vi "DQBuf.vi"(0 "nInputHandle":u64, 2 "nTimeOut":u32, 5 "error in (no error)":errorcluster) -> (14 "nOutputHandle":u64, 15 "ImgBuf":u8[](array[numeric]), 16 "ppFrameBuffer":u64, 17 "Dst":T1, 18 "GX_STATUS":i32, 19 "error out":errorcluster)   [LabVIEW 2016, in "GxLVLib.lvlib"]
uses:
  GxLVLib.lvlib
  GxIAPI.dll
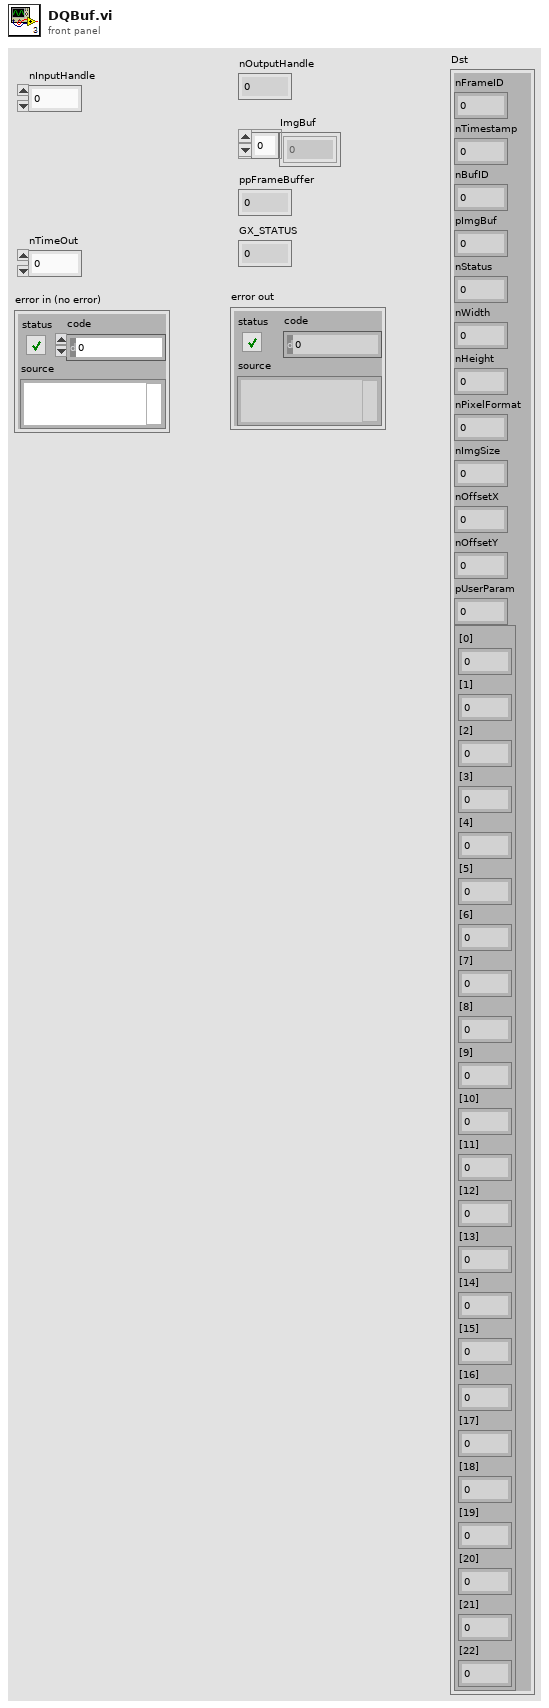
[diagram p1: front panel]
types:
  T1 = cluster{"nFrameID":u64, "nTimestamp":u64, "nBufID":u64, "pImgBuf":u64, "nStatus":i32, "nWidth":i32, "nHeight":i32, "nPixelFormat":i32, "nImgSize":i32, "nOffsetX":i32, "nOffsetY":i32, "pUserParam":i32, cluster{"[0]":i32, "[1]":i32, "[2]":i32, "[3]":i32, "[4]":i32, "[5]":i32, "[6]":i32, "[7]":i32, "[8]":i32, "[9]":i32, "[10]":i32, "[11]":i32, "[12]":i32, "[13]":i32, "[14]":i32, "[15]":i32, "[16]":i32, "[17]":i32, "[18]":i32, "[19]":i32, "[20]":i32, "[21]":i32, "[22]":i32}}
  T2 = cluster{"[0]":i32, "[1]":i32, "[2]":i32, "[3]":i32, "[4]":i32, "[5]":i32, "[6]":i32, "[7]":i32, "[8]":i32, "[9]":i32, "[10]":i32, "[11]":i32, "[12]":i32, "[13]":i32, "[14]":i32, "[15]":i32, "[16]":i32, "[17]":i32, "[18]":i32, "[19]":i32, "[20]":i32, "[21]":i32, "[22]":i32}
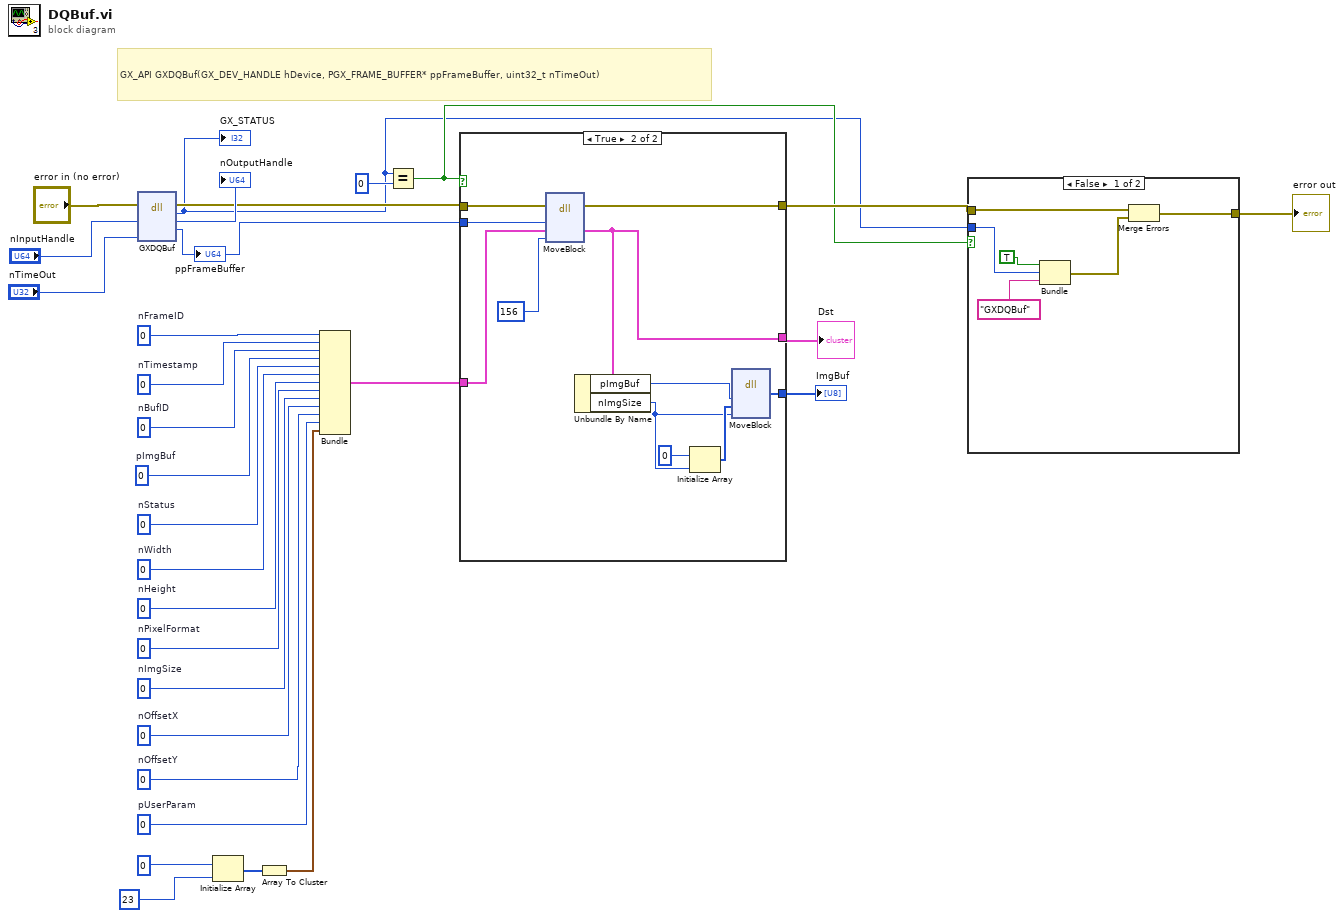
[diagram p0: block diagram]
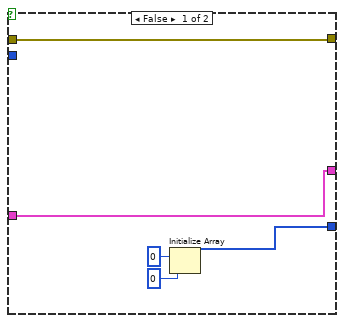
[diagram p2: hidden frame]
diagram:
  w9 = u64 0  # pImgBuf
  w14 = 0  # pUserParam
  w15 = 0  # nOffsetY
  w16 = 0  # nOffsetX
  w17 = 0  # nImgSize
  w18 = 0  # nPixelFormat
  w19 = 0  # nHeight
  w20 = 0  # nWidth
  w21 = 0  # nStatus
  w22 = u64 0  # nBufID
  w23 = u64 0  # nTimestamp
  w24 = u64 0  # nFrameID
  # "GX_API GXDQBuf(GX_DEV_HANDLE hDevice, PGX_FRAME_BUFFER* ppFrameBuffer, uint32_t nTimeOut)"
  n1 = dll-call lib="GxIAPI.dll" fn="GXDQBuf"(error in="error in (no error)", "phDevice"="nInputHandle", "nTimeOut"="nTimeOut") -> (error out=w8:errorcluster, "GX_STATUS"=w1:i32, "phDevice"=→"nOutputHandle":i64, "ppFrameBuffer"=w7:u64)  [unwired: 4 in, 1 out]
  "GX_STATUS" <- w1
  "ppFrameBuffer" <- w7
  n2 = Initialize Array(0, 23) -> (w11:i32[])
  n3 = Array To Cluster(array=w11) -> (cluster=w10:T2)
  n4 = Bundle("nFrameID"=w24, "nTimestamp"=w23, "nBufID"=w22, "pImgBuf"=w9, "nStatus"=w21, "nWidth"=w20, "nHeight"=w19, "nPixelFormat"=w18, "nImgSize"=w17, "nOffsetX"=w16, "nOffsetY"=w15, "pUserParam"=w14, w10) -> (w6:T1)  [unwired: 1 in]
  n5 = Equal?(x=w1, y=0) -> (x = y?=w2:bool)
  n6 = case shown="True" w2 {
    tunnel: w8 -> [w31 w45]
    tunnel: w7 -> [_ w44]
    tunnel: w6 -> [w35 w43]
    tunnel: [w35 w39] -> w5
    tunnel: [w32 w38] -> w4
    tunnel: [w31 w37] -> w3
    frame False {
      n7 = Initialize Array(u8 0 ("element"), 0 ("dimension size")) -> (w32:u8[])
    }
    frame True {
      n8 = dll-call lib="LabVIEW" fn="MoveBlock"(error in=w45, "Src"=w44, "Dst"=w43, "size"=156) -> (error out=w37:errorcluster, "Dst"=w39:T1)  [unwired: 5 in, 1 out]
      n9 = Unbundle By Name(w39) -> ("pImgBuf"=w41:u64, "nImgSize"=w36:i32)
      n10 = Initialize Array(u8 0, w36) -> (w42:u8[])
      n11 = dll-call lib="LabVIEW" fn="MoveBlock"("Src"=w41, "Dst"=w42, "size"=w36) -> ("Dst"=w38:u8[])  [unwired: 6 in, 2 out]
    }
  }
  "Dst" <- w5
  "ImgBuf" <- w4
  n12 = case shown="False" w2 {
    tunnel: w3 -> [w52 w53]
    tunnel: [w51 w53] -> w28
    tunnel: w1 -> [w49 _]
    frame False {
      n13 = Bundle(TRUE, "GX_STATUS"=w49, "GXDQBuf") -> (w50:cluster{bool, "GX_STATUS":i32, string})  [unwired: 1 in]
      n14 = Merge Errors(w52, w50) -> (w51:errorcluster)
    }
    frame True {
    }
  }
  "error out" <- w28
